vi "3.3.3.-Capas RGB y HSV en Imagen.vi"(9 "UMBRAL":dbl(knob) scale=0.0..255.0, 10 "CAPA DE COLOR":T1) -> (3 "IMAGEN BINARIZADA":picture)   [LabVIEW 2020]
uses:
  3.3.0.-ENUM Capas RGB a HSV.ctl
panel:
  in  "Seleccionar Imagen":path
  # "Visión Artificial - Extraer Capas RGB y HSV\nDiego Cervantes Rodríguez\ndicer0.com"
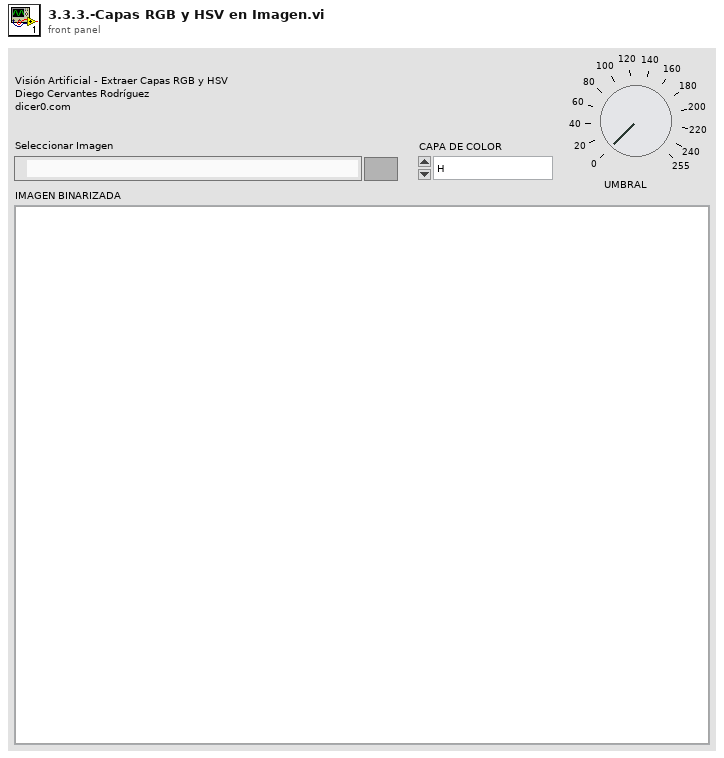
[diagram p1: front panel]
types:
  T1 = typedef "3.3.0.-ENUM Capas RGB a HSV.ctl" = enum16{"H", "S", "V", "R", "G", "B", "RGB2GRAY MATLAB"}
  T2 = typedef "imagedata.ctl" = cluster{"image type":i32, "image depth":i32, "image":u8[], "mask":u8[], "colors":u32[], "Rectangle":cluster{"left":i16, "top":i16, "right":i16, "bottom":i16}}
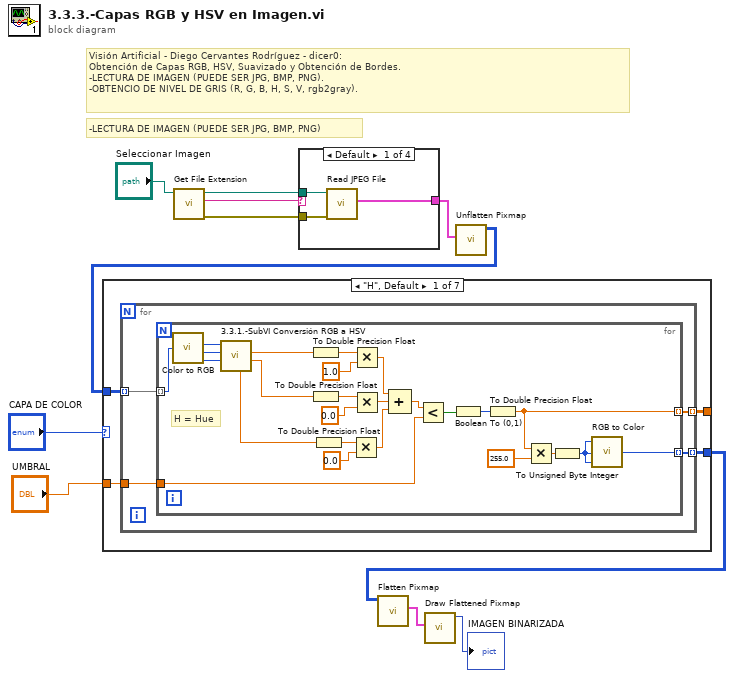
[diagram p0: block diagram]
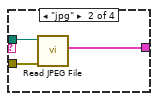
[diagram p2: hidden frame]
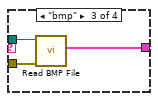
[diagram p3: hidden frame]
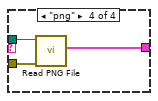
[diagram p4: hidden frame]
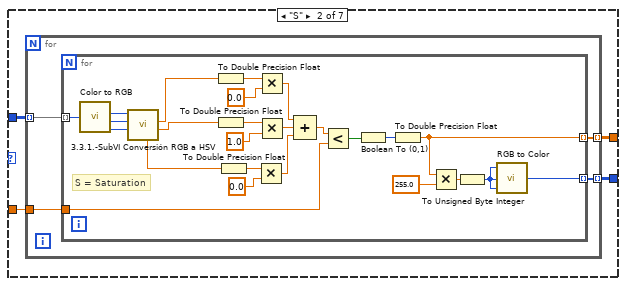
[diagram p5: hidden frame]
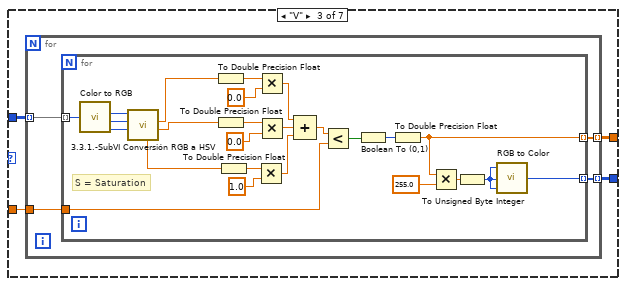
[diagram p6: hidden frame]
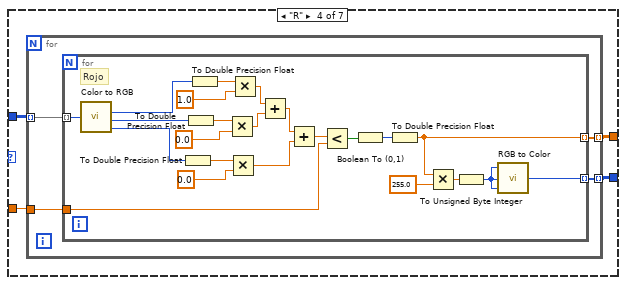
[diagram p7: hidden frame]
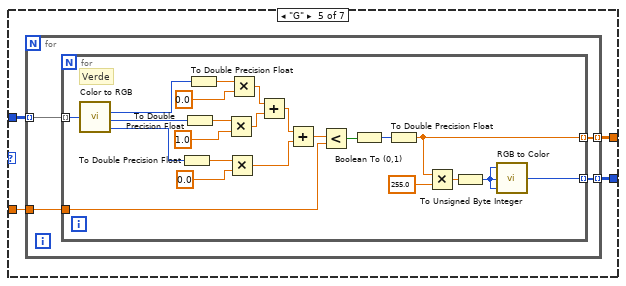
[diagram p8: hidden frame]
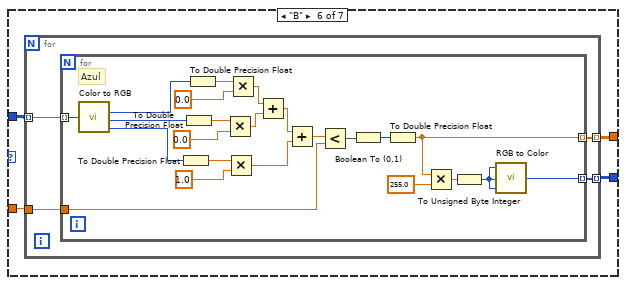
[diagram p9: hidden frame]
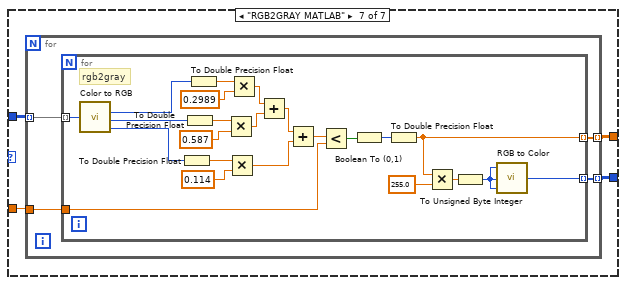
[diagram p10: hidden frame]
diagram:
  # "-LECTURA DE IMAGEN (PUEDE SER JPG, BMP, PNG)"
  # "Visión Artificial - Diego Cervantes Rodríguez - dicer0: \nObtención de Capas RGB, HSV, Suavizado y Obtención de Bordes.\n-LECTURA DE IMAGEN (PUEDE SER JPG, BMP, PNG).\n-OBTENCIO DE NIVEL DE GRIS (R, G, B, H, S, V, rgb2gray)."
  n1 = call <vilib>:"Get File Extension.vi"("file"="Seleccionar Imagen") -> ("error out"=w5:errorcluster, "lowercase file extension"=w3:string, "dup file"=w4:path)  [unwired: 6 in, 2 out]
  n2 = case shown="Default" w3 {
    tunnel: w4 -> [w14 w17 w20 w23]
    tunnel: w5 -> [w13 w16 w19 w22]
    tunnel: [w12 w15 w18 w21] -> w1
    frame Default {
      n3 = call <vilib>:"Read JPEG File.vi"("error in (no error)"=w13, "path to JPEG file"=w14) -> ("image data"=w12:T2)  [unwired: 7 in, 2 out]
    }
    frame "jpg" {
      n4 = call <vilib>:"Read JPEG File.vi"("error in (no error)"=w16, "path to JPEG file"=w17) -> ("image data"=w15:T2)  [unwired: 7 in, 2 out]
    }
    frame "bmp" {
      n5 = call <vilib>:"Read BMP File.vi"("error in (no error)"=w19, "path to BMP file"=w20) -> ("image data"=w18:T2)  [unwired: 7 in, 2 out]
    }
    frame "png" {
      n6 = call <vilib>:"Read PNG File.vi"("error in (no error)"=w22, "path to PNG file"=w23) -> ("image data"=w21:T2)  [unwired: 7 in, 2 out]
    }
  }
  n7 = call <vilib>:"Unflatten Pixmap.vi"("image data"=w1) -> ("24-bit pixmap"=w11:u32[][])  [unwired: 4 in, 6 out]
  n8 = case shown="\"H\", Default" "CAPA DE COLOR" {
    tunnel: [w27 w58 w93 w124 w155 w186 w217] -> _
    tunnel: [w26 w57 w92 w123 w154 w185 w216] -> w8
    tunnel: "UMBRAL" -> [w24 w59 w91 w125 w156 w187 w218]
    tunnel: w11 -> [w25 w60 w90 w126 w157 w188 w219]
    frame "H", Default {
      n9 = for {
        tunnel: w25 -> [w31] mode=indexing
        tunnel: [w30] -> w27 mode=indexing
        tunnel: [w29] -> w26 mode=indexing
        tunnel: w24 -> [w28]
        n10 = for {
          tunnel: w31 -> [w56] mode=indexing
          tunnel: [w50] -> w30 mode=indexing
          tunnel: [w46] -> w29 mode=indexing
          tunnel: w28 -> [w42]
          # "H = Hue"
          n11 = call <vilib>:"Color to RGB.vi"("Color"=w56) -> ("R"=w37:u8, "G"=w36:u8, "B"=w35:u8)  [unwired: 1 out]
          n12 = call "3.3.1.-SubVI Conversión RGB a HSV.vi"("B"=w35, "G"=w36, "R"=w37) -> ("S"=w33:dbl, "H"=w34:dbl, "V"=w32:dbl)  [unwired: 6 in]
          n13 = To Double Precision Float(number=w34) -> (double precision float=w45:dbl)
          n14 = To Double Precision Float(number=w33) -> (double precision float=w44:dbl)
          n15 = To Double Precision Float(number=w32) -> (double precision float=w43:dbl)
          n16 = Multiply(x=w43, y=0.0) -> (x*y=w39:dbl)
          n17 = Multiply(x=w45, y=1.0) -> (x*y=w41:dbl)
          n18 = Multiply(x=w44, y=0.0) -> (x*y=w40:dbl)
          n19 = Compound Arithmetic op=ADD(w41, w40, w39) -> (w38:dbl)
          n20 = Less?(x=w38, y=w42) -> (x < y?=w52:bool)
          n21 = Boolean To (0,1)(Boolean=w52) -> (0, 1=w51:i16)
          n22 = To Double Precision Float(number=w51) -> (double precision float=w50:dbl)
          n23 = Multiply(x=w50, y=255.0) -> (x*y=w48:dbl)
          n24 = To Unsigned Byte Integer(number=w48) -> (unsigned 8bit integer=w47:u8)
          n25 = call <vilib>:"RGB to Color.vi"("B"=w47, "G"=w47, "R"=w47) -> ("Color"=w46:u32)
        }
      }
    }
    frame "S" {
      n26 = for {
        tunnel: w60 -> [w64] mode=indexing
        tunnel: [w63] -> w58 mode=indexing
        tunnel: [w62] -> w57 mode=indexing
        tunnel: w59 -> [w61]
        n27 = for {
          tunnel: w64 -> [w89] mode=indexing
          tunnel: [w83] -> w63 mode=indexing
          tunnel: [w79] -> w62 mode=indexing
          tunnel: w61 -> [w75]
          # "S = Saturation"
          n28 = call <vilib>:"Color to RGB.vi"("Color"=w89) -> ("R"=w70:u8, "G"=w69:u8, "B"=w68:u8)  [unwired: 1 out]
          n29 = call "3.3.1.-SubVI Conversión RGB a HSV.vi"("B"=w68, "G"=w69, "R"=w70) -> ("S"=w66:dbl, "H"=w67:dbl, "V"=w65:dbl)  [unwired: 6 in]
          n30 = To Double Precision Float(number=w67) -> (double precision float=w78:dbl)
          n31 = To Double Precision Float(number=w66) -> (double precision float=w77:dbl)
          n32 = To Double Precision Float(number=w65) -> (double precision float=w76:dbl)
          n33 = Multiply(x=w76, y=0.0) -> (x*y=w72:dbl)
          n34 = Multiply(x=w78, y=0.0) -> (x*y=w74:dbl)
          n35 = Multiply(x=w77, y=1.0) -> (x*y=w73:dbl)
          n36 = Compound Arithmetic op=ADD(w74, w73, w72) -> (w71:dbl)
          n37 = Less?(x=w71, y=w75) -> (x < y?=w85:bool)
          n38 = Boolean To (0,1)(Boolean=w85) -> (0, 1=w84:i16)
          n39 = To Double Precision Float(number=w84) -> (double precision float=w83:dbl)
          n40 = Multiply(x=w83, y=255.0) -> (x*y=w81:dbl)
          n41 = To Unsigned Byte Integer(number=w81) -> (unsigned 8bit integer=w80:u8)
          n42 = call <vilib>:"RGB to Color.vi"("B"=w80, "G"=w80, "R"=w80) -> ("Color"=w79:u32)
        }
      }
    }
    frame "V" {
      n43 = for {
        tunnel: w90 -> [w97] mode=indexing
        tunnel: [w96] -> w93 mode=indexing
        tunnel: [w95] -> w92 mode=indexing
        tunnel: w91 -> [w94]
        n44 = for {
          tunnel: w97 -> [w122] mode=indexing
          tunnel: [w116] -> w96 mode=indexing
          tunnel: [w112] -> w95 mode=indexing
          tunnel: w94 -> [w108]
          # "S = Saturation"
          n45 = call <vilib>:"Color to RGB.vi"("Color"=w122) -> ("R"=w103:u8, "G"=w102:u8, "B"=w101:u8)  [unwired: 1 out]
          n46 = call "3.3.1.-SubVI Conversión RGB a HSV.vi"("B"=w101, "G"=w102, "R"=w103) -> ("S"=w99:dbl, "H"=w100:dbl, "V"=w98:dbl)  [unwired: 6 in]
          n47 = To Double Precision Float(number=w100) -> (double precision float=w111:dbl)
          n48 = To Double Precision Float(number=w99) -> (double precision float=w110:dbl)
          n49 = To Double Precision Float(number=w98) -> (double precision float=w109:dbl)
          n50 = Multiply(x=w109, y=1.0) -> (x*y=w105:dbl)
          n51 = Multiply(x=w111, y=0.0) -> (x*y=w107:dbl)
          n52 = Multiply(x=w110, y=0.0) -> (x*y=w106:dbl)
          n53 = Compound Arithmetic op=ADD(w107, w106, w105) -> (w104:dbl)
          n54 = Less?(x=w104, y=w108) -> (x < y?=w118:bool)
          n55 = Boolean To (0,1)(Boolean=w118) -> (0, 1=w117:i16)
          n56 = To Double Precision Float(number=w117) -> (double precision float=w116:dbl)
          n57 = Multiply(x=w116, y=255.0) -> (x*y=w114:dbl)
          n58 = To Unsigned Byte Integer(number=w114) -> (unsigned 8bit integer=w113:u8)
          n59 = call <vilib>:"RGB to Color.vi"("B"=w113, "G"=w113, "R"=w113) -> ("Color"=w112:u32)
        }
      }
    }
    frame "R" {
      n60 = for {
        tunnel: w126 -> [w130] mode=indexing
        tunnel: [w129] -> w124 mode=indexing
        tunnel: [w128] -> w123 mode=indexing
        tunnel: w125 -> [w127]
        n61 = for {
          tunnel: w130 -> [w153] mode=indexing
          tunnel: [w147] -> w129 mode=indexing
          tunnel: [w143] -> w128 mode=indexing
          tunnel: w127 -> [w136]
          # "Rojo"
          n62 = call <vilib>:"Color to RGB.vi"("Color"=w153) -> ("R"=w142:u8, "G"=w140:u8, "B"=w138:u8)  [unwired: 1 out]
          n63 = To Double Precision Float(number=w138) -> (double precision float=w137:dbl)
          n64 = To Double Precision Float(number=w140) -> (double precision float=w139:dbl)
          n65 = To Double Precision Float(number=w142) -> (double precision float=w141:dbl)
          n66 = Multiply(x=w139, y=0.0) -> (x*y=w133:dbl)
          n67 = Multiply(x=w137, y=0.0) -> (x*y=w134:dbl)
          n68 = Multiply(x=w141, y=1.0) -> (x*y=w132:dbl)
          n69 = Add(x=w132, y=w133) -> (x+y=w135:dbl)
          n70 = Add(x=w135, y=w134) -> (x+y=w131:dbl)
          n71 = Less?(x=w131, y=w136) -> (x < y?=w149:bool)
          n72 = Boolean To (0,1)(Boolean=w149) -> (0, 1=w148:i16)
          n73 = To Double Precision Float(number=w148) -> (double precision float=w147:dbl)
          n74 = Multiply(x=w147, y=255.0) -> (x*y=w145:dbl)
          n75 = To Unsigned Byte Integer(number=w145) -> (unsigned 8bit integer=w144:u8)
          n76 = call <vilib>:"RGB to Color.vi"("B"=w144, "G"=w144, "R"=w144) -> ("Color"=w143:u32)
        }
      }
    }
    frame "G" {
      n77 = for {
        tunnel: w157 -> [w161] mode=indexing
        tunnel: [w160] -> w155 mode=indexing
        tunnel: [w159] -> w154 mode=indexing
        tunnel: w156 -> [w158]
        n78 = for {
          tunnel: w161 -> [w184] mode=indexing
          tunnel: [w178] -> w160 mode=indexing
          tunnel: [w174] -> w159 mode=indexing
          tunnel: w158 -> [w167]
          # "Verde"
          n79 = call <vilib>:"Color to RGB.vi"("Color"=w184) -> ("R"=w173:u8, "G"=w171:u8, "B"=w169:u8)  [unwired: 1 out]
          n80 = To Double Precision Float(number=w169) -> (double precision float=w168:dbl)
          n81 = To Double Precision Float(number=w171) -> (double precision float=w170:dbl)
          n82 = To Double Precision Float(number=w173) -> (double precision float=w172:dbl)
          n83 = Multiply(x=w170, y=1.0) -> (x*y=w164:dbl)
          n84 = Multiply(x=w168, y=0.0) -> (x*y=w165:dbl)
          n85 = Multiply(x=w172, y=0.0) -> (x*y=w163:dbl)
          n86 = Add(x=w163, y=w164) -> (x+y=w166:dbl)
          n87 = Add(x=w166, y=w165) -> (x+y=w162:dbl)
          n88 = Less?(x=w162, y=w167) -> (x < y?=w180:bool)
          n89 = Boolean To (0,1)(Boolean=w180) -> (0, 1=w179:i16)
          n90 = To Double Precision Float(number=w179) -> (double precision float=w178:dbl)
          n91 = Multiply(x=w178, y=255.0) -> (x*y=w176:dbl)
          n92 = To Unsigned Byte Integer(number=w176) -> (unsigned 8bit integer=w175:u8)
          n93 = call <vilib>:"RGB to Color.vi"("B"=w175, "G"=w175, "R"=w175) -> ("Color"=w174:u32)
        }
      }
    }
    frame "B" {
      n94 = for {
        tunnel: w188 -> [w192] mode=indexing
        tunnel: [w191] -> w186 mode=indexing
        tunnel: [w190] -> w185 mode=indexing
        tunnel: w187 -> [w189]
        n95 = for {
          tunnel: w192 -> [w215] mode=indexing
          tunnel: [w209] -> w191 mode=indexing
          tunnel: [w205] -> w190 mode=indexing
          tunnel: w189 -> [w198]
          # "Azul"
          n96 = call <vilib>:"Color to RGB.vi"("Color"=w215) -> ("R"=w204:u8, "G"=w202:u8, "B"=w200:u8)  [unwired: 1 out]
          n97 = To Double Precision Float(number=w200) -> (double precision float=w199:dbl)
          n98 = To Double Precision Float(number=w202) -> (double precision float=w201:dbl)
          n99 = To Double Precision Float(number=w204) -> (double precision float=w203:dbl)
          n100 = Multiply(x=w201, y=0.0) -> (x*y=w195:dbl)
          n101 = Multiply(x=w199, y=1.0) -> (x*y=w196:dbl)
          n102 = Multiply(x=w203, y=0.0) -> (x*y=w194:dbl)
          n103 = Add(x=w194, y=w195) -> (x+y=w197:dbl)
          n104 = Add(x=w197, y=w196) -> (x+y=w193:dbl)
          n105 = Less?(x=w193, y=w198) -> (x < y?=w211:bool)
          n106 = Boolean To (0,1)(Boolean=w211) -> (0, 1=w210:i16)
          n107 = To Double Precision Float(number=w210) -> (double precision float=w209:dbl)
          n108 = Multiply(x=w209, y=255.0) -> (x*y=w207:dbl)
          n109 = To Unsigned Byte Integer(number=w207) -> (unsigned 8bit integer=w206:u8)
          n110 = call <vilib>:"RGB to Color.vi"("B"=w206, "G"=w206, "R"=w206) -> ("Color"=w205:u32)
        }
      }
    }
    frame "RGB2GRAY MATLAB" {
      n111 = for {
        tunnel: w219 -> [w223] mode=indexing
        tunnel: [w222] -> w217 mode=indexing
        tunnel: [w221] -> w216 mode=indexing
        tunnel: w218 -> [w220]
        n112 = for {
          tunnel: w223 -> [w246] mode=indexing
          tunnel: [w240] -> w222 mode=indexing
          tunnel: [w236] -> w221 mode=indexing
          tunnel: w220 -> [w229]
          # "rgb2gray"
          n113 = call <vilib>:"Color to RGB.vi"("Color"=w246) -> ("R"=w235:u8, "G"=w233:u8, "B"=w231:u8)  [unwired: 1 out]
          n114 = To Double Precision Float(number=w231) -> (double precision float=w230:dbl)
          n115 = To Double Precision Float(number=w233) -> (double precision float=w232:dbl)
          n116 = To Double Precision Float(number=w235) -> (double precision float=w234:dbl)
          n117 = Multiply(x=w232, y=0.587) -> (x*y=w226:dbl)
          n118 = Multiply(x=w230, y=0.114) -> (x*y=w227:dbl)
          n119 = Multiply(x=w234, y=0.2989) -> (x*y=w225:dbl)
          n120 = Add(x=w225, y=w226) -> (x+y=w228:dbl)
          n121 = Add(x=w228, y=w227) -> (x+y=w224:dbl)
          n122 = Less?(x=w224, y=w229) -> (x < y?=w242:bool)
          n123 = Boolean To (0,1)(Boolean=w242) -> (0, 1=w241:i16)
          n124 = To Double Precision Float(number=w241) -> (double precision float=w240:dbl)
          n125 = Multiply(x=w240, y=255.0) -> (x*y=w238:dbl)
          n126 = To Unsigned Byte Integer(number=w238) -> (unsigned 8bit integer=w237:u8)
          n127 = call <vilib>:"RGB to Color.vi"("B"=w237, "G"=w237, "R"=w237) -> ("Color"=w236:u32)
        }
      }
    }
  }
  n128 = call <vilib>:"Flatten Pixmap.vi"("24-bit pixmap"=w8) -> ("image data"=w9:T2)  [unwired: 10 in]
  n129 = call <vilib>:"Draw Flattened Pixmap.vi"("image data"=w9) -> ("new picture"=→"IMAGEN BINARIZADA":picture)  [unwired: 8 in]
